vi "MAIN.vi"() -> ()   [LabVIEW 2015]
uses:
  <vilib>/Analysis/7linalg.llb/Solve Linear Equations (single right hand).vi
  <vilib>/Analysis/baseanly.llb/Solve Linear Equations By Cholesky.vi
  <vilib>/Analysis/baseanly.llb/Real Matrix to Compact Array.vi
  <vilib>/Analysis/baseanly.llb/Real Compact Tri-Matrix Linear Eqs.vi
  <vilib>/Analysis/7linalg.llb/Solve Linear Eqs (General).vi
  <vilib>/Analysis/7linalg.llb/Solve Linear Eqs (Gen, single right hand).vi
  <vilib>/Analysis/NI_AALPro.lvlib
  <vilib>/gmath/NI_Gmath.lvlib
panel:
  in  "Next":bool
  out "Graph":cluster{dbl[], dbl[]}[](graph)=[{[3.0, 49.0, 69.0, 90.0, 98.0, 99.0], [69.0, 10.0, 18.0, 60.0, 46.0, 88.0]}, {[20.751196172248846, 59.49760765550242, 75.25837320574166, 95.46889952153109, 98.86602870813394], [44.60925039872407, -0.21850079744815593, 32.26475279106858, 63.15948963317382, 47.09728867623602]}, {[38.50239234449758, 62.74162679425834, 84.53110047846891, 97.13397129186606, 98.93301435406697], [20.218500797448154, 3.735247208931419, 56.84051036682618, 44.90271132376398, 67.54864433811801]}, {array[5005 elements], array[5005 elements]}, {array[9601 elements], array[9601 elements]}]
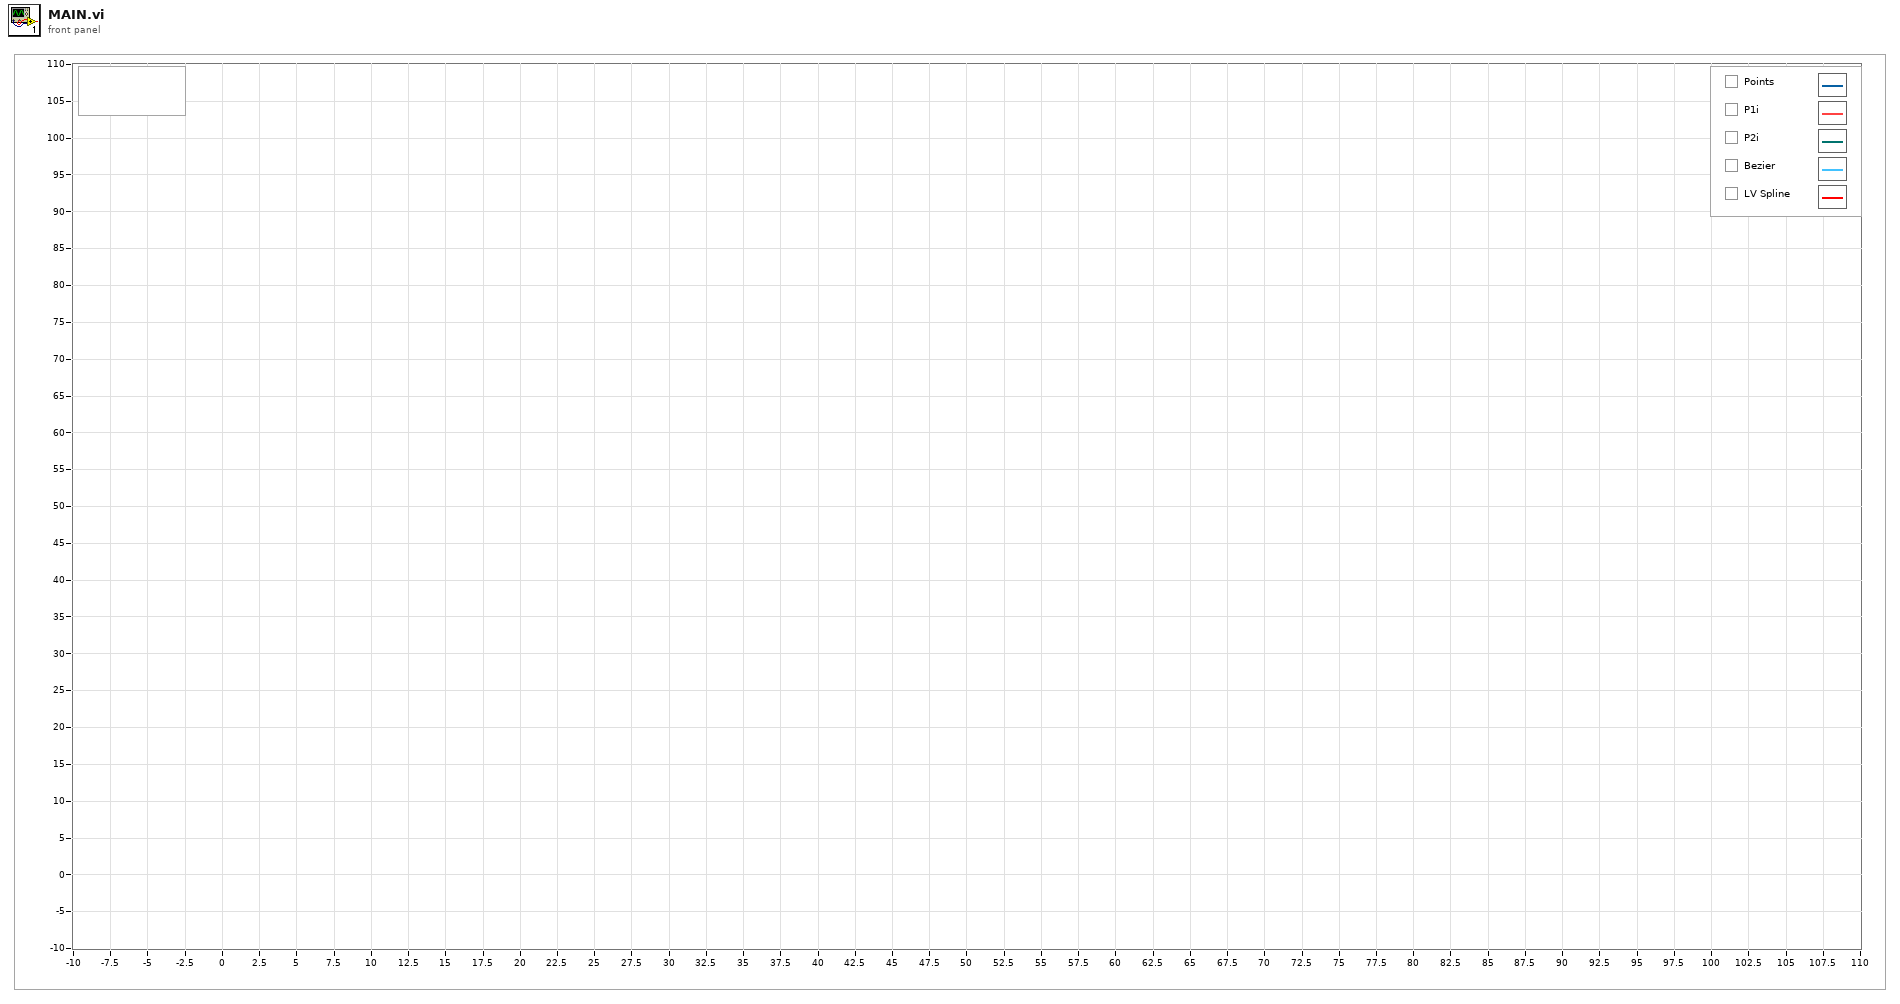
[diagram p1: front panel]
types:
  T1 = typedef "NI_Matrix.lvlib/RealMatrix.ctl" = dbl[][]
  T2 = cluster{"Solution Vector":dbl[], "Solution Vector":dbl[]}
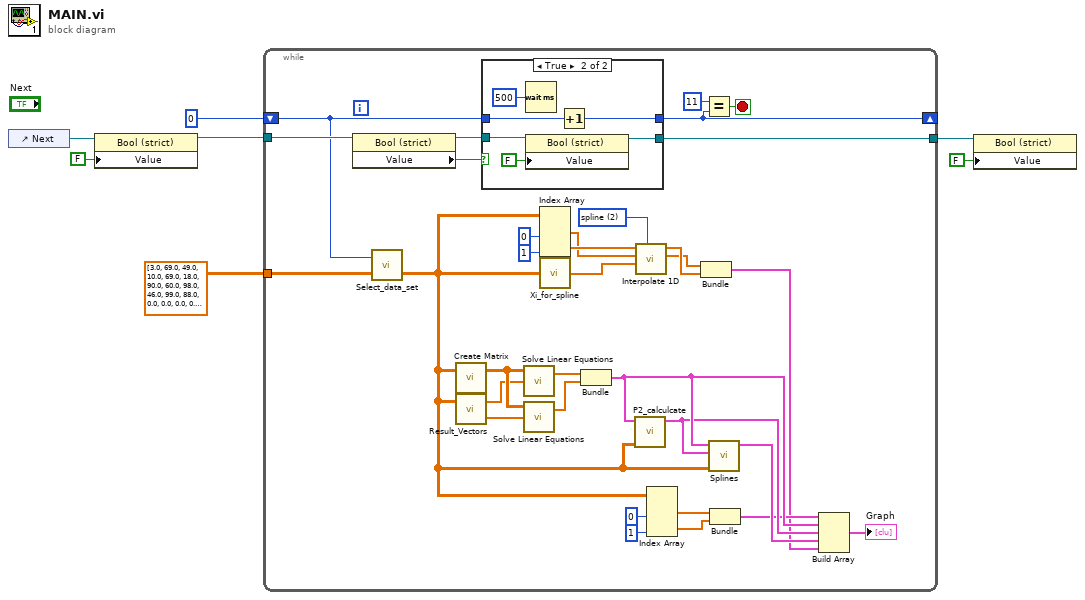
[diagram p0: block diagram]
diagram:
  n1 = control-ref of="Next"() -> (w7:refnum<vi>)
  n2 = property class="Bool (strict)"(reference=w7, "Value"=FALSE) -> (reference out=w5:refnum<vi>)  [unwired: 1 in, 1 out]
  n3 = while {
    tunnel: w5 -> [w17]
    tunnel: [w14] -> w2
    tunnel: dbl[][][] [[[3.0, 69.0], [49.0, 10.0], [69.0, 18.0], [90.0, 60.0], [98.0, 46.0], [99.0, 88.0], [0.0, 0.0], [0.0, 0.0], [0.0, 0.0], [0.0, 0.0], [0.0, 0.0], [0.0, 0.0], [0.0, 0.0], [0.0, 0.0], [0.0, 0.0], [0.0, 0.0], [0.0, 0.0], [0.0, 0.0], [0.0, 0.0], [0.0, 0.0], [0.0, 0.0], [0.0, 0.0], [0.0, 0.0], [0.0, 0.0], [0.0, 0.0], [0.0, 0.0], [0.0, 0.0], [0.0, 0.0], [0.0, 0.0], [0.0, 0.0], [0.0, 0.0], [0.0, 0.0], [0.0, 0.0], [0.0, 0.0], [0.0, 0.0], [0.0, 0.0], [0.0, 0.0], [0.0, 0.0], [0.0, 0.0], [0.0, 0.0], [0.0, 0.0], [0.0, 0.0], [0.0, 0.0], [0.0, 0.0], [0.0, 0.0], [0.0, 0.0]], [[81.0, 17.0], [28.0, 80.0], [8.0, 71.0], [26.0, 16.0], [55.0, 12.0], [99.0, 14.0], [0.0, 0.0], [0.0, 0.0], [0.0, 0.0], [0.0, 0.0], [0.0, 0.0], [0.0, 0.0], [0.0, 0.0], [0.0, 0.0], [0.0, 0.0], [0.0, 0.0], [0.0, 0.0], [0.0, 0.0], [0.0, 0.0], [0.0, 0.0], [0.0, 0.0], [0.0, 0.0], [0.0, 0.0], [0.0, 0.0], [0.0, 0.0], [0.0, 0.0], [0.0, 0.0], [0.0, 0.0], [0.0, 0.0], [0.0, 0.0], [0.0, 0.0], [0.0, 0.0], [0.0, 0.0], [0.0, 0.0], [0.0, 0.0], [0.0, 0.0], [0.0, 0.0], [0.0, 0.0], [0.0, 0.0], [0.0, 0.0], [0.0, 0.0], [0.0, 0.0], [0.0, 0.0], [0.0, 0.0], [0.0, 0.0], [0.0, 0.0]], [[50.0, 31.0], [46.0, 46.0], [5.0, 44.0], [8.0, 33.0], [22.0, 73.0], [41.0, 60.0], [0.0, 0.0], [0.0, 0.0], [0.0, 0.0], [0.0, 0.0], [0.0, 0.0], [0.0, 0.0], [0.0, 0.0], [0.0, 0.0], [0.0, 0.0], [0.0, 0.0], [0.0, 0.0], [0.0, 0.0], [0.0, 0.0], [0.0, 0.0], [0.0, 0.0], [0.0, 0.0], [0.0, 0.0], [0.0, 0.0], [0.0, 0.0], [0.0, 0.0], [0.0, 0.0], [0.0, 0.0], [0.0, 0.0], [0.0, 0.0], [0.0, 0.0], [0.0, 0.0], [0.0, 0.0], [0.0, 0.0], [0.0, 0.0], [0.0, 0.0], [0.0, 0.0], [0.0, 0.0], [0.0, 0.0], [0.0, 0.0], [0.0, 0.0], [0.0, 0.0], [0.0, 0.0], [0.0, 0.0], [0.0, 0.0], [0.0, 0.0]], [[5.0, 54.0], [23.0, 85.0], [48.0, 87.0], [91.0, 49.0], [92.0, 93.0], [98.0, 89.0], [0.0, 0.0], [0.0, 0.0], [0.0, 0.0], [0.0, 0.0], [0.0, 0.0], [0.0, 0.0], [0.0, 0.0], [0.0, 0.0], [0.0, 0.0], [0.0, 0.0], [0.0, 0.0], [0.0, 0.0], [0.0, 0.0], [0.0, 0.0], [0.0, 0.0], [0.0, 0.0], [0.0, 0.0], [0.0, 0.0], [0.0, 0.0], [0.0, 0.0], [0.0, 0.0], [0.0, 0.0], [0.0, 0.0], [0.0, 0.0], [0.0, 0.0], [0.0, 0.0], [0.0, 0.0], [0.0, 0.0], [0.0, 0.0], [0.0, 0.0], [0.0, 0.0], [0.0, 0.0], [0.0, 0.0], [0.0, 0.0], [0.0, 0.0], [0.0, 0.0], [0.0, 0.0], [0.0, 0.0], [0.0, 0.0], [0.0, 0.0]], [[6.0, 86.0], [13.0, 73.0], [24.0, 50.0], [39.0, 52.0], [58.0, 86.0], [85.0, 2.0], [0.0, 0.0], [0.0, 0.0], [0.0, 0.0], [0.0, 0.0], [0.0, 0.0], [0.0, 0.0], [0.0, 0.0], [0.0, 0.0], [0.0, 0.0], [0.0, 0.0], [0.0, 0.0], [0.0, 0.0], [0.0, 0.0], [0.0, 0.0], [0.0, 0.0], [0.0, 0.0], [0.0, 0.0], [0.0, 0.0], [0.0, 0.0], [0.0, 0.0], [0.0, 0.0], [0.0, 0.0], [0.0, 0.0], [0.0, 0.0], [0.0, 0.0], [0.0, 0.0], [0.0, 0.0], [0.0, 0.0], [0.0, 0.0], [0.0, 0.0], [0.0, 0.0], [0.0, 0.0], [0.0, 0.0], [0.0, 0.0], [0.0, 0.0], [0.0, 0.0], [0.0, 0.0], [0.0, 0.0], [0.0, 0.0], [0.0, 0.0]], [[36.0, 39.0], [39.0, 13.0], [39.0, 70.0], [48.0, 30.0], [72.0, 46.0], [94.0, 87.0], [0.0, 0.0], [0.0, 0.0], [0.0, 0.0], [0.0, 0.0], [0.0, 0.0], [0.0, 0.0], [0.0, 0.0], [0.0, 0.0], [0.0, 0.0], [0.0, 0.0], [0.0, 0.0], [0.0, 0.0], [0.0, 0.0], [0.0, 0.0], [0.0, 0.0], [0.0, 0.0], [0.0, 0.0], [0.0, 0.0], [0.0, 0.0], [0.0, 0.0], [0.0, 0.0], [0.0, 0.0], [0.0, 0.0], [0.0, 0.0], [0.0, 0.0], [0.0, 0.0], [0.0, 0.0], [0.0, 0.0], [0.0, 0.0], [0.0, 0.0], [0.0, 0.0], [0.0, 0.0], [0.0, 0.0], [0.0, 0.0], [0.0, 0.0], [0.0, 0.0], [0.0, 0.0], [0.0, 0.0], [0.0, 0.0], [0.0, 0.0]], [[36.75570504584947, 41.180339887498945], [44.02113032590307, 31.18033988749895], [44.02113032590307, 18.819660112501055], [36.75570504584947, 8.819660112501055], [25.000000000000004, 5.0], [13.24429495415054, 8.819660112501047], [5.978869674096931, 18.819660112501047], [5.978869674096927, 31.180339887498945], [13.244294954150533, 41.180339887498945], [24.999999999999996, 45.0], [36.75570504584947, 41.180339887498945], [0.0, 0.0], [0.0, 0.0], [0.0, 0.0], [0.0, 0.0], [0.0, 0.0], [0.0, 0.0], [0.0, 0.0], [0.0, 0.0], [0.0, 0.0], [0.0, 0.0], [0.0, 0.0], [0.0, 0.0], [0.0, 0.0], [0.0, 0.0], [0.0, 0.0], [0.0, 0.0], [0.0, 0.0], [0.0, 0.0], [0.0, 0.0], [0.0, 0.0], [0.0, 0.0], [0.0, 0.0], [0.0, 0.0], [0.0, 0.0], [0.0, 0.0], [0.0, 0.0], [0.0, 0.0], [0.0, 0.0], [0.0, 0.0], [0.0, 0.0], [0.0, 0.0], [0.0, 0.0], [0.0, 0.0], [0.0, 0.0], [0.0, 0.0]], [[0.0, 0.0], [20.0, 0.0], [20.0, 50.0], [40.0, 50.0], [40.0, 0.0], [60.0, 0.0], [0.0, 0.0], [0.0, 0.0], [0.0, 0.0], [0.0, 0.0], [0.0, 0.0], [0.0, 0.0], [0.0, 0.0], [0.0, 0.0], [0.0, 0.0], [0.0, 0.0], [0.0, 0.0], [0.0, 0.0], [0.0, 0.0], [0.0, 0.0], [0.0, 0.0], [0.0, 0.0], [0.0, 0.0], [0.0, 0.0], [0.0, 0.0], [0.0, 0.0], [0.0, 0.0], [0.0, 0.0], [0.0, 0.0], [0.0, 0.0], [0.0, 0.0], [0.0, 0.0], [0.0, 0.0], [0.0, 0.0], [0.0, 0.0], [0.0, 0.0], [0.0, 0.0], [0.0, 0.0], [0.0, 0.0], [0.0, 0.0], [0.0, 0.0], [0.0, 0.0], [0.0, 0.0], [0.0, 0.0], [0.0, 0.0], [0.0, 0.0]], [[0.0, 0.0], [10.0, 0.0], [20.0, 0.0], [20.0, 25.0], [20.0, 50.0], [30.0, 50.0], [40.0, 50.0], [40.0, 25.0], [40.0, 0.0], [50.0, 0.0], [0.0, 0.0], [0.0, 0.0], [0.0, 0.0], [0.0, 0.0], [0.0, 0.0], [0.0, 0.0], [0.0, 0.0], [0.0, 0.0], [0.0, 0.0], [0.0, 0.0], [0.0, 0.0], [0.0, 0.0], [0.0, 0.0], [0.0, 0.0], [0.0, 0.0], [0.0, 0.0], [0.0, 0.0], [0.0, 0.0], [0.0, 0.0], [0.0, 0.0], [0.0, 0.0], [0.0, 0.0], [0.0, 0.0], [0.0, 0.0], [0.0, 0.0], [0.0, 0.0], [0.0, 0.0], [0.0, 0.0], [0.0, 0.0], [0.0, 0.0], [0.0, 0.0], [0.0, 0.0], [0.0, 0.0], [0.0, 0.0], [0.0, 0.0], [0.0, 0.0]], [[0.0, 0.0], [5.0, 0.0], [10.0, 0.0], [15.0, 0.0], [20.0, 0.0], [20.0, 10.0], [20.0, 20.0], [20.0, 30.0], [20.0, 40.0], [25.0, 40.0], [30.0, 40.0], [35.0, 40.0], [40.0, 40.0], [40.0, 30.0], [40.0, 20.0], [40.0, 10.0], [40.0, 0.0], [45.0, 0.0], [50.0, 0.0], [0.0, 0.0], [0.0, 0.0], [0.0, 0.0], [0.0, 0.0], [0.0, 0.0], [0.0, 0.0], [0.0, 0.0], [0.0, 0.0], [0.0, 0.0], [0.0, 0.0], [0.0, 0.0], [0.0, 0.0], [0.0, 0.0], [0.0, 0.0], [0.0, 0.0], [0.0, 0.0], [0.0, 0.0], [0.0, 0.0], [0.0, 0.0], [0.0, 0.0], [0.0, 0.0], [0.0, 0.0], [0.0, 0.0], [0.0, 0.0], [0.0, 0.0], [0.0, 0.0], [0.0, 0.0]], [[0.0, 0.0], [2.0, 0.0], [4.0, 0.0], [6.0, 0.0], [8.0, 0.0], [10.0, 0.0], [12.0, 0.0], [14.0, 0.0], [16.0, 0.0], [18.0, 0.0], [20.0, 0.0], [20.0, 4.0], [20.0, 8.0], [20.0, 12.0], [20.0, 16.0], [20.0, 20.0], [20.0, 24.0], [20.0, 28.0], [20.0, 32.0], [20.0, 36.0], [20.0, 40.0], [22.0, 40.0], [24.0, 40.0], [26.0, 40.0], [28.0, 40.0], [30.0, 40.0], [32.0, 40.0], [34.0, 40.0], [36.0, 40.0], [38.0, 40.0], [40.0, 40.0], [40.0, 36.0], [40.0, 32.0], [40.0, 28.0], [40.0, 24.0], [40.0, 20.0], [40.0, 16.0], [40.0, 12.0], [40.0, 8.0], [40.0, 4.0], [40.0, 0.0], [42.0, 0.0], [44.0, 0.0], [46.0, 0.0], [48.0, 0.0], [50.0, 0.0]]] ("output array") -> [w12]
    shift-right: [w8] -> _
    shift-left: 0 -> [w10]
    stop <- w13 stop-if-true
    w19 = 2 items=["nearest", "linear", "spline", "cubic Hermite", "Lagrange"] ("method")
    n4 = property class="Bool (strict)"(reference=w17) -> (reference out=w15:refnum<vi>, "Value"=w16:bool)  [unwired: 1 in, 1 out]
    n5 = call "Select_data_set.vi"("array"=w12, "index"=w10) -> ("Array 2"=w11:dbl[][])  [unwired: 1 in]
    n6 = call "Create Matrix.vi"("Array"=w11) -> ("Real Matrix"=w37:T1)  [unwired: 2 in]
    n7 = call "Result_Vectors.vi"("Array"=w11) -> ("Y-vector"=w35:dbl[], "X-vector"=w36:dbl[])  [unwired: 1 in]
    n8 = case shown="True" w16 {
      tunnel: w15 -> [w42 w48]
      tunnel: [w42 w46] -> w14
      tunnel: w10 -> [w41 w45]
      tunnel: [w41 w44] -> w8
      frame False {
      }
      frame True {
        n9 = Wait (ms)(milliseconds to wait=u32 500) -> ()  [unwired: 1 out]
        n10 = property class="Bool (strict)"(reference=w48, "Value"=FALSE) -> (reference out=w46:refnum<vi>)  [unwired: 1 in, 1 out]
        n11 = Increment(x=w45) -> (x+1=w44:i32)
      }
    }
    n12 = call-poly <vilib>:"Solve Linear Equations.vi"("Known Vector"=w36, "Input Matrix"=w37) -> ("Solution Vector"=w28:dbl[])  [unwired: 1 in, 1 out]
    n13 = call-poly <vilib>:"Solve Linear Equations.vi"("Known Vector"=w35, "Input Matrix"=w37) -> ("Solution Vector"=w27:dbl[])  [unwired: 1 in, 1 out]
    n14 = Index Array(array=w11, index (col) #1=0 ("disabled index (col)"), index (col) #2=1 ("index (col)")) -> (element #1=w23:dbl[], element #2=w24:dbl[])  [unwired: 2 in]
    n15 = call "Xi_for_spline.vi"("Array"=w11) -> ("Xi"=w18:dbl[])
    n16 = Bundle("Solution Vector"=w28, "Solution Vector"=w27) -> (w33:T2)  [unwired: 1 in]
    n17 = call "P2_calculcate.vi"("Points"=w11, "P1i"=w33) -> ("P2i"=w32:cluster{dbl[], dbl[]})  [unwired: 9 in]
    n18 = call <vilib>:"Interpolate 1D.vi"("method"=w19, "xi"=w18, "X"=w23, "Y"=w24) -> ("xi used"=w21:dbl[], "yi"=w22:dbl[])  [unwired: 5 in, 1 out]
    n19 = Index Array(array=w11, index (col) #1=0 ("disabled index (col)"), index (col) #2=1 ("index (col)")) -> (element #1=w30:dbl[], element #2=w29:dbl[])  [unwired: 2 in]
    n20 = Bundle("xi used"=w21, "yi"=w22) -> (w20:cluster{"xi used":dbl[], "yi":dbl[]})  [unwired: 1 in]
    n21 = Equal?(x=11 ("y"), y=w8) -> (x = y?=w13:bool)
    n22 = call "Splines.vi"("Points"=w11, "P2i"=w32, "P1i"=w33) -> ("Spline"=w34:cluster{dbl[], dbl[]})  [unwired: 8 in]
    n23 = Bundle("Array 2"=w30, "Array 2"=w29) -> (w31:cluster{"Array 2":dbl[], "Array 2":dbl[]})  [unwired: 1 in]
    n24 = Build Array(w31, w33, w32, w34, w20) -> (→"Graph":cluster{"xi used":dbl[], "yi":dbl[]}[])
  }
  n25 = property class="Bool (strict)"(reference=w2, "Value"=FALSE) -> ()  [unwired: 1 in, 2 out]
